vi "Reset.vi"(8 "error in (no error)":errorcluster, 11 "VISA resource name":refnum<visa-resource-name>) -> (0 "error out":errorcluster, 3 "VISA resource name out":refnum<visa-resource-name>)   [LabVIEW 2025]
doc: "Resets the instrument and then sends a set of default setup commands to the instrument."
uses:
  <vilib>/Instr/_visa.llb/VISA Flush IO Buffer Mask.ctl
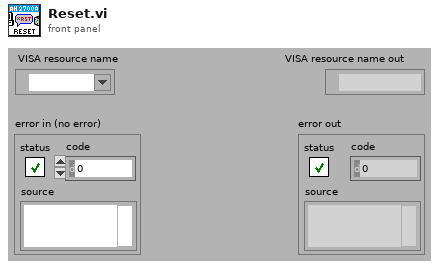
[diagram p1: front panel]
types:
  T1 = typedef "VISA Flush IO Buffer Mask.ctl" = u16
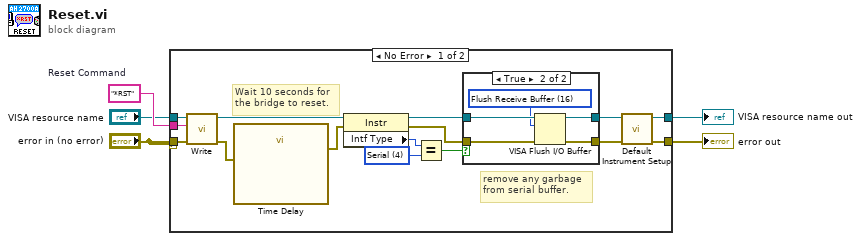
[diagram p0: block diagram]
diagram:
  w5 = "*RST"  # Reset Command
  n1 = case shown="No Error" "error in (no error)" {
    selector: "error in (no error)" -> [_ w29]
    tunnel: "error in (no error)" -> [w20 _]
    tunnel: w5 -> [w19 _]
    tunnel: "VISA resource name" -> [w18 w28]
    tunnel: [w16 w28] -> w3
    tunnel: [w15 w29] -> w2
    frame No Error {
      w14 = u16 4 items=["GPIB"=1, "VXI"=2, "GPIB-VXI"=3, "Serial"=4, "PXI"=5, "TCPIP"=6, "USB"=7, "FireWire"=9] ("Interface Information:Interface Type")
      # "remove any garbage\nfrom serial buffer."
      # "Wait 10 seconds for\nthe bridge to reset."
      n2 = call "Write.vi"("error in"=w20, "command"=w19, "VISA resource name"=w18) -> ("error out"=w17:errorcluster, "VISA resource name out"=w12:refnum<visa-resource-name>)  [unwired: 7 in]
      n3 = call "Time Delay"("error in (no error)"=w17) -> ("error out"=w11:errorcluster)  [unwired: 10 in]
      n4 = property class="Instr"(reference=w12, error in=w11) -> (reference out=w9:refnum<visa-resource-name>, error out=w8:errorcluster, "Intf Type"=w13:u16)
      n5 = Equal?(x=w13, y=w14) -> (x = y?=w6:bool)
      n6 = case shown="True" w6 {
        tunnel: [w22 w27] -> w10
        tunnel: w9 -> [w22 w26]
        tunnel: w8 -> [w21 w25]
        tunnel: [w21 w24] -> w7
        frame False {
        }
        frame True {
          w23 = T1 16 items=["Flush Receive Buffer"=16, "Write Transmit Buffer to Device"=32, "Flush Receive Buffer (No I/O)"=64, "Flush Transmit Buffer"=128] ("Mask")
          n7 = VISA Flush I/O Buffer(VISA resource name=w26, mask (16)=w23, error in (no error)=w25) -> (VISA resource name out=w27:refnum<visa-resource-name>, error out=w24:errorcluster)
        }
      }
      n8 = call "Default Instrument Setup.vi"("error in (no error)"=w7, "VISA resource name"=w10) -> ("error out"=w15:errorcluster, "VISA resource name out"=w16:refnum<visa-resource-name>)  [unwired: 8 in]
    }
    frame Error {
    }
  }
  "error out" <- w2
  "VISA resource name out" <- w3
